vi "Start DAQ.vi"(8 "error in (no error)":errorcluster, 11 "PID in":refnum<class "INL PID.lvclass">) -> (0 "error out":errorcluster, 3 "PID out":refnum<class "INL PID.lvclass">)   [LabVIEW 2011, in "INL PID.lvclass"]
uses:
  INL PID.lvclass
  INL PID.lvclass/INL PID.ctl
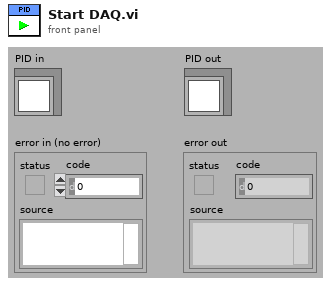
[diagram p1: front panel]
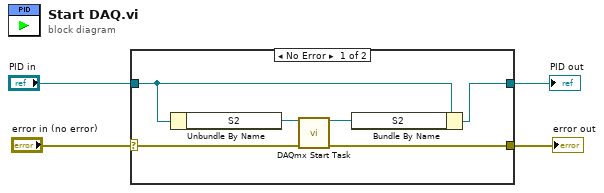
[diagram p0: block diagram]
diagram:
  n1 = case shown="No Error" "error in (no error)" {
    selector: "error in (no error)" -> [w9 w12]
    tunnel: [w6 w12] -> w3
    tunnel: [w5 w11] -> w1
    tunnel: "PID in" -> [w8 w11]
    frame No Error {
      n2 = Unbundle By Name(w8) -> ("S2"=w10:refnum<k21>)
      n3 = call <vilib>:"DAQmx Start Task.vi"("task/channels in"=w10, "error in"=w9) -> ("task out"=w7:refnum<k21>, "error out"=w6:errorcluster)  [unwired: 12 in]
      n4 = Bundle By Name(cluster=w8, "S2"=w7) -> (w5:refnum<class "INL PID.lvclass">)
    }
    frame Error {
    }
  }
  "error out" <- w3
  "PID out" <- w1
